vi "Shutdown Complete.vi"(8 "error in":errorcluster, 10 "Shutdown Complete":bool, 11 "SCADA in":refnum<class "EMS.lvclass">) -> (0 "error out":errorcluster, 3 "SCADA out":refnum<class "EMS.lvclass">)   [LabVIEW 2018, in "EMS Core.lvlib" / "EMS.lvclass"]
uses:
  EMS.lvclass
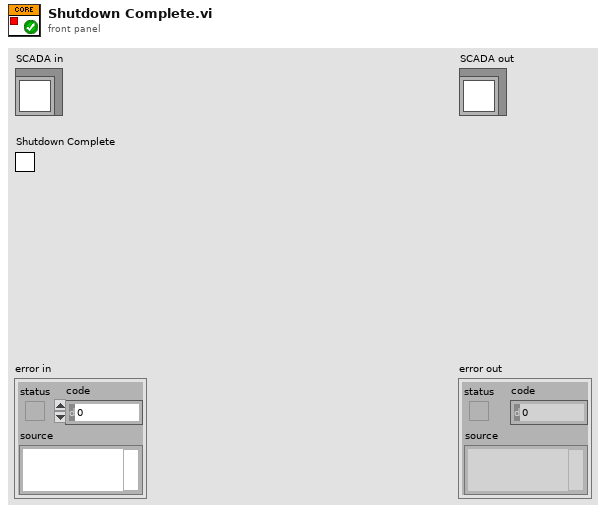
[diagram p1: front panel]
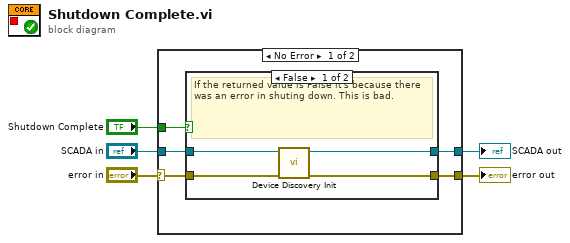
[diagram p0: block diagram]
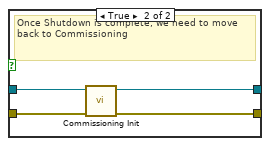
[diagram p2: hidden frame]
diagram:
  n1 = case shown="No Error" "error in" {
    selector: "error in" -> [w7 w20]
    tunnel: [w6 w20] -> w4
    tunnel: [w8 w19] -> w2
    tunnel: "SCADA in" -> [w9 w19]
    tunnel: "Shutdown Complete" -> [w10 _]
    frame No Error {
      n2 = case shown="False" w10 {
        tunnel: w9 -> [w14 w18]
        tunnel: [w13 w15] -> w8
        tunnel: w7 -> [w11 w17]
        tunnel: [w12 w16] -> w6
        frame False {
          # "If the returned value is False it's because there was an error in shuting down. This is bad."
          n3 = call "Device Discovery Init.vi"("error in"=w11, "SCADA in"=w14) -> ("error out"=w12:errorcluster, "SCADA out"=w13:refnum<class "EMS.lvclass">)  [unwired: 8 in]
        }
        frame True {
          # "Once Shutdown is complete, we need to move back to Commissioning"
          n4 = call "Commissioning Init.vi"("error in"=w17, "SCADA in"=w18) -> ("error out"=w16:errorcluster, "SCADA out"=w15:refnum<class "EMS.lvclass">)  [unwired: 8 in]
        }
      }
    }
    frame Error {
    }
  }
  "error out" <- w4
  "SCADA out" <- w2
